vi "Read from DI DB_byRef.vi"(8 "error in (no error)":errorcluster, 9 "Length (-1)":i32=-1, 10 "Modbus Address":u16, 11 "Cache Ref in":refnum<data-value>) -> (0 "error out":errorcluster, 2 "Values":bool[](array[boolean]), 3 "Cache Ref out":refnum<data-value>)   [LabVIEW 2018]
uses:
  MB Data Block.lvclass
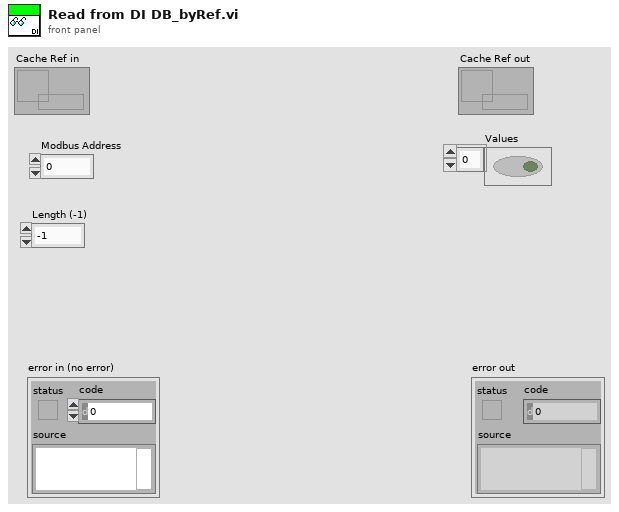
[diagram p1: front panel]
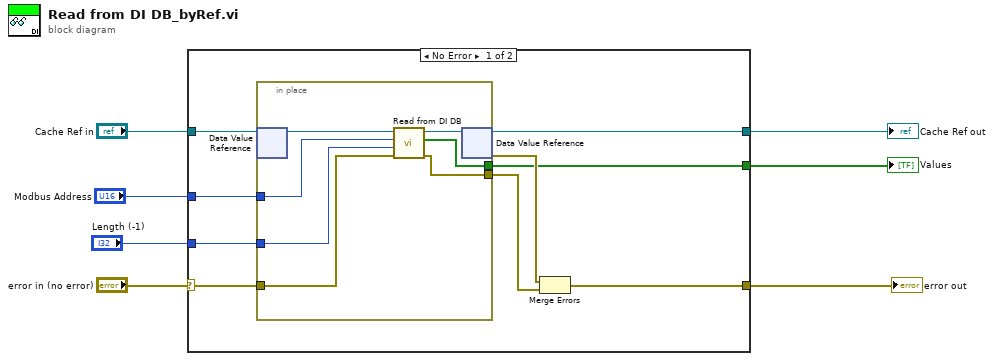
[diagram p0: block diagram]
diagram:
  n1 = case shown="No Error" "error in (no error)" {
    selector: "error in (no error)" -> [w10 w25]
    tunnel: "Cache Ref in" -> [w16 w24]
    tunnel: [w15 w24] -> w6
    tunnel: "Modbus Address" -> [w14 _]
    tunnel: [w11 w25] -> w4
    tunnel: [w9 _] -> w2
    tunnel: "Length (-1)" -> [w8 _]
    frame No Error {
      n2 = in-place {
        in-place-border: w10 -> [w20]
        in-place-border: [w21] -> w13
        in-place-border: w14 -> [w19]
        in-place-border: [w18] -> w9
        in-place-border: w8 -> [w17]
        n3 = in-place-dvr #1(w16) -> (w23:refnum<class "MB Data Block.lvclass">)  [unwired: 1 out]
        n4 = call-dynamic "Read from DI DB.vi"("error in (no error)"=w20, "Length (-1)"=w17, "Modbus Address"=w19, "MB Data Block in"=w23) -> ("error out"=w21:errorcluster, "Data out"=w18:bool[], "MB Data Block out"=w22:refnum<class "MB Data Block.lvclass">)  [unwired: 5 in]
        n5 = in-place-dvr #1(w22) -> (w15:refnum<data-value>, w12:errorcluster)
      }
      n6 = Merge Errors(w12, w13) -> (w11:errorcluster)
    }
    frame Error {
    }
  }
  "error out" <- w4
  "Cache Ref out" <- w6
  "Values" <- w2
